vi "Init Data.vi"(10 "Data":T1 {"Time Stamp" format="%<%x %.3X>T"}) -> (3 "Msg out":refnum<class "Msg.lvclass">)   [LabVIEW 2023, in "ConstellationCommand.lvlib" / "Msg.lvclass"]
uses:
  Msg.lvclass
  Msg.lvclass/Msg.ctl
  Data.ctl
  ConstellationCommand.lvlib
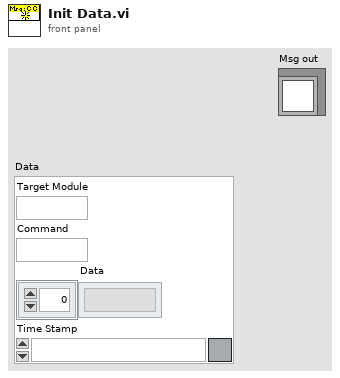
[diagram p1: front panel]
types:
  T1 = typedef "ConstellationCommand.lvlib/Data.ctl" = cluster{"Target Module":string, "Command":string, "Data":string[], "Time Stamp":timestamp}
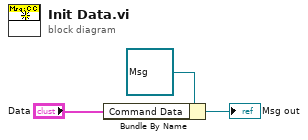
[diagram p0: block diagram]
diagram:
  n1 = Bundle By Name(cluster=refnum<class "Msg.lvclass"> refnum ("ConstellationCommand.lvlib:Msg.lvclass"), "Command Data"="Data") -> (→"Msg out":refnum<class "Msg.lvclass">)
